vi "Configure_Graph_Y1.vi"(8 "error in (no error)":errorcluster, 10 "Y1 Axis Settings":T1={"Y1 axis"="Id", "MINIMUM"=-1e-05, "MAXIMUM"=0.0, "LIN or LOG axis"="LIN"} {"MAXIMUM" format="%.2e"; "MINIMUM" format="%_2e"}, 11 "VISA In":refnum<visa-resource-name>) -> (0 "error out":errorcluster, 3 "VISA Out":refnum<visa-resource-name>)   [LabVIEW 2012]
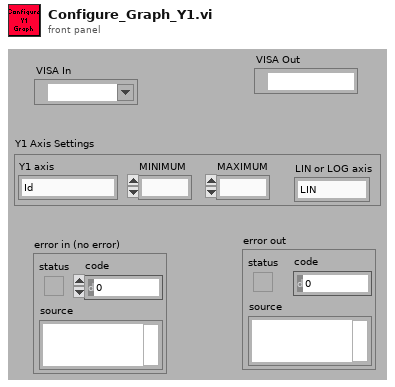
[diagram p1: front panel]
types:
  T1 = cluster{"Y1 axis":string, "MINIMUM":ext, "MAXIMUM":ext, "LIN or LOG axis":string}
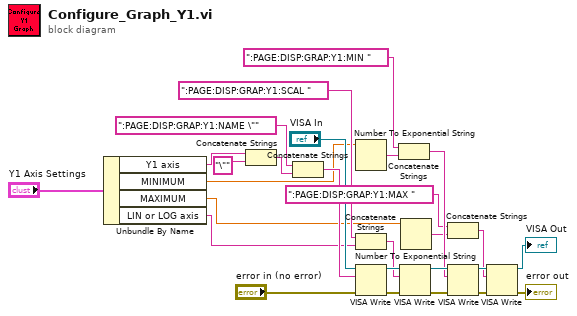
[diagram p0: block diagram]
diagram:
  n1 = Unbundle By Name("Y1 Axis Settings") -> ("Y1 axis"=w2:string, "MINIMUM"=w3:ext, "MAXIMUM"=w4:ext, "LIN or LOG axis"=w1:string)
  n2 = Concatenate Strings(w2, "\"" ("string")) -> (w25:string)
  n3 = Concatenate Strings(":PAGE:DISP:GRAP:Y1:NAME \"" ("write buffer"), w25) -> (w23:string)
  n4 = Number To Exponential String(number=w3) -> (E-format string=w13:string)  [unwired: 3 in]
  n5 = Concatenate Strings(":PAGE:DISP:GRAP:Y1:SCAL " ("write buffer"), w1) -> (w15:string)
  n6 = VISA Write(VISA resource name="VISA In", write buffer=w23, error in (no error)="error in (no error)") -> (VISA resource name out=w22:refnum<visa-resource-name>, error out=w19:errorcluster)  [unwired: 1 out]
  n7 = Concatenate Strings(":PAGE:DISP:GRAP:Y1:MIN " ("write buffer"), w13) -> (w12:string)
  n8 = VISA Write(VISA resource name=w22, write buffer=w15, error in (no error)=w19) -> (VISA resource name out=w21:refnum<visa-resource-name>, error out=w18:errorcluster)  [unwired: 1 out]
  n9 = Number To Exponential String(number=w4) -> (E-format string=w11:string)  [unwired: 3 in]
  n10 = Concatenate Strings(":PAGE:DISP:GRAP:Y1:MAX " ("write buffer"), w11) -> (w9:string)
  n11 = VISA Write(VISA resource name=w21, write buffer=w12, error in (no error)=w18) -> (VISA resource name out=w20:refnum<visa-resource-name>, error out=w17:errorcluster)  [unwired: 1 out]
  n12 = VISA Write(VISA resource name=w20, write buffer=w9, error in (no error)=w17) -> (VISA resource name out=→"VISA Out":refnum<visa-resource-name>, error out=→"error out":errorcluster)  [unwired: 1 out]
